vi "test1-ModuleCreatedDestroyed_Queue.vi"(8 "error in (no error)":errorcluster, 11 "TestCase in":refnum<class "testcase-CSMGlobalLog.lvclass">) -> (0 "error out":errorcluster, 3 "TestCase out":refnum<class "testcase-CSMGlobalLog.lvclass">)   [LabVIEW 2017, in "testcase-CSMGlobalLog.lvclass"]
uses:
  testcase-CSMGlobalLog.lvclass
  testcase-CSMGlobalLog.lvclass/testcase-CSMGlobalLog.ctl
  64b6e408-f0cd-4aee-a387-1a6bb95babb2.vi
  <vilib>/addons/_JKI Toolkits/VI Tester/TestCase.llb/TestCase.lvclass
  src/user.lib/_NEVSTOP/Communicable State Machine(CSM)/Utility/Periodic String Filter Setting.ctl
  src/user.lib/_NEVSTOP/Communicable State Machine(CSM)/Communicable State Machine.lvlib
  C:/Program Files (x86)/National Instruments/LabVIEW 2017/vi.lib/addons/_JKI Toolkits/VI Tester/TestCase.llb/TestCase.lvclass
panel:
  out "String Cache Each Loop":string
  out "String cache total":string
  out "LoopCount":i32
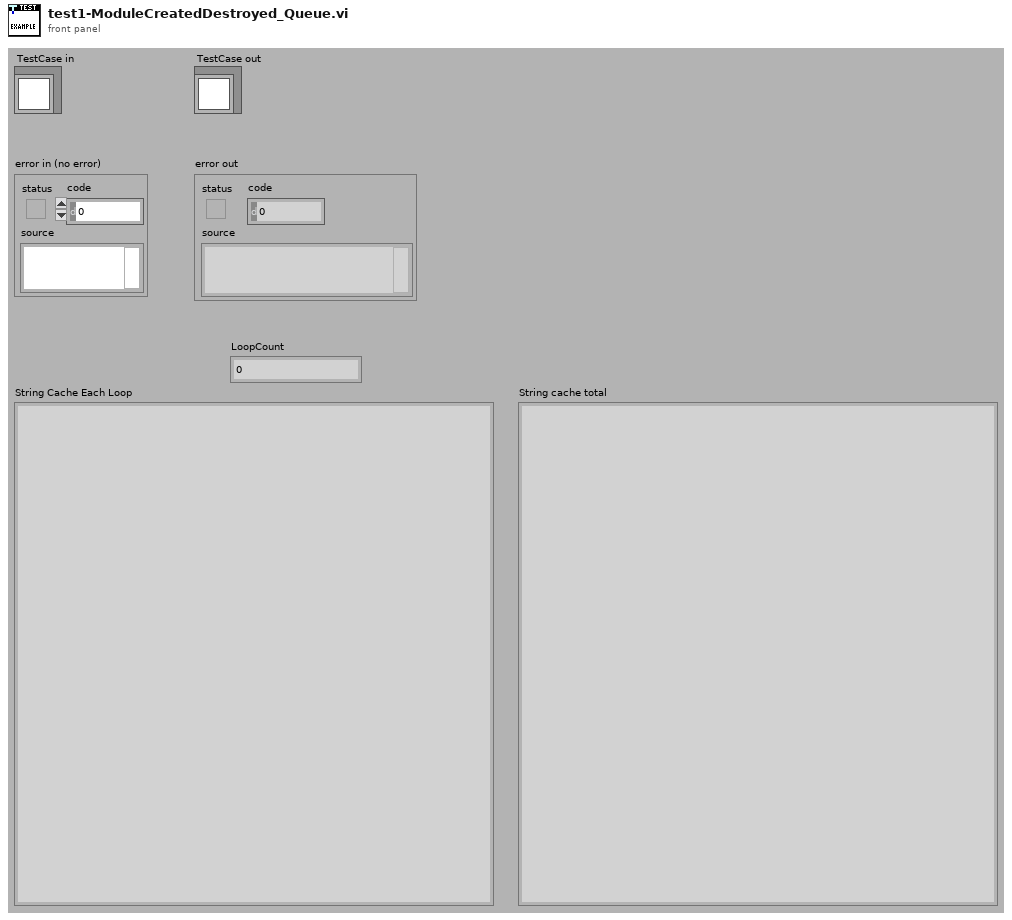
[diagram p1: front panel]
types:
  T1 = typedef "Communicable State Machine.lvlib/Periodic String Filter Setting.ctl" = cluster{"threashold(#/s)":dbl, "Check Peroid(s)":dbl}
  T2 = typedef "Communicable State Machine.lvlib/_CSM_GlobalLog_MSG.ctl" = cluster{"Name (\"\" to Use UUID)":string, "Current State":string, "Arguments":string, "Source Message":T3, "Source Module":string, "Complete(T)/Start(F)":bool, "LogType":T4, "Time Stamp":timestamp}
  T3 = typedef "Communicable State Machine.lvlib/_CSM_Response Source Message.ctl" = cluster{"‘State":string, "’Arguments":string, "’Error":errorcluster}
  T4 = typedef "Communicable State Machine.lvlib/_CSM_GlobalLog_MSG_TYPE.ctl" = enum16{"User Log", "State Change", "Status", "Interrupt", "Register", "Unregister", "Error Log", "Module Created", "Module Destroyed", "Async Message", "No-Rep Async Message", "Sync Message", "AsyncMsg Complete", "SyncMsg Complete"}
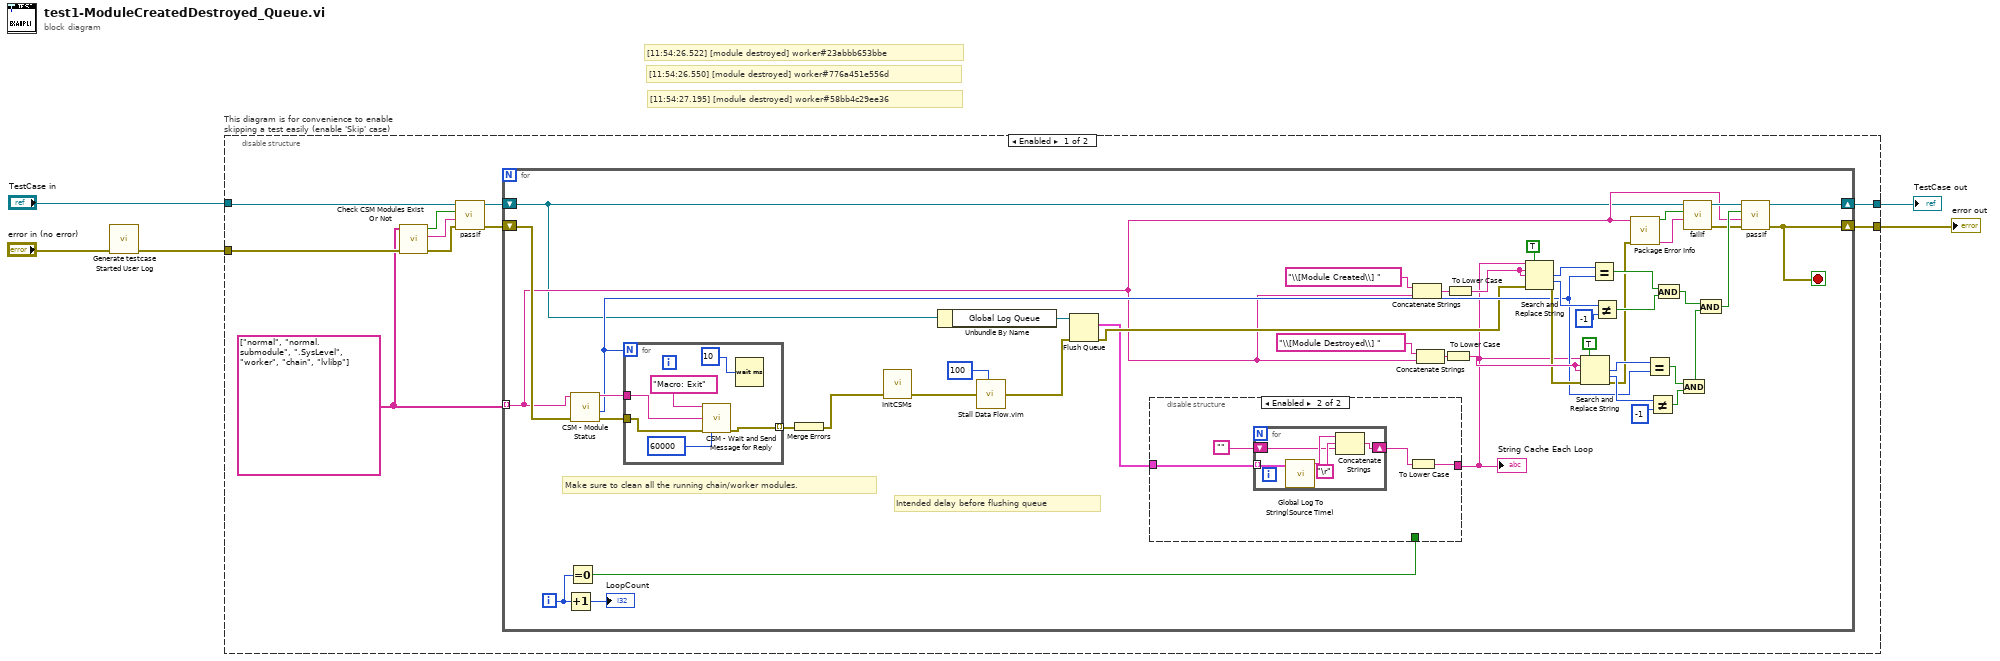
[diagram p0: block diagram]
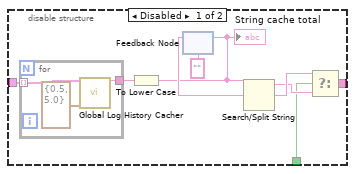
[diagram p2: hidden frame]
diagram:
  # "[11:54:26.522] [module destroyed] worker#23abbb653bbe"
  # "[11:54:27.195] [module destroyed] worker#58bb4c29ee36"
  # "[11:54:26.550] [module destroyed] worker#776a451e556d"
  n1 = call "Generate testcase Started User Log.vi"("Error In"="error in (no error)") -> ("error out"=w1:errorcluster)  [unwired: 10 in]
  n2 = disable-structure "This diagram is for convenience to enable skipping a test easily (enable 'Skip' case)" shown="Enabled" {
    disable-tunnel: "TestCase in" -> [w10 w93]
    disable-tunnel: [w14 w91] -> w2
    disable-tunnel: [w15 w92] -> w4
    disable-tunnel: w1 -> [w8 w90]
    frame Enabled {
      w6 = string[] ["normal", "normal.submodule", ".SysLevel", "worker", "chain", "lvlibp"]
      n3 = call "Check CSM Modules Exist Or Not.vi"("error in"=w8, "CSM names in"=w6) -> ("error out"=w11:errorcluster, "Debug string"=w12:string, "All Modules Exist?"=w13:bool)  [unwired: 7 in]
      n4 = call-dynamic "passIf.vi"("error in (no error)"=w11, "message (\"\")"=w12, "pass"=w13, "TestCase in"=w10) -> ("error out"=w7:errorcluster, "TestCase out"=w9:refnum<class "testcase-CSMGlobalLog.lvclass">)  [unwired: 6 in]
      n5 = for {
        tunnel: w6 -> [w17] mode=indexing
        shift-right: [w32] -> w15
        shift-left: w7 -> [w24]
        shift-right: [w62] -> w14
        shift-left: w9 -> [w16]
        i -> [w26]
        stop <- w32 stop-if-true
        # "Intended delay before flushing queue"
        # "Make sure to clean all the running chain/worker modules."
        n6 = Increment(x=w26) -> (x+1=→"LoopCount":i32)
        n7 = Equal To 0?(x=w26) -> (x = 0?=w25:bool)
        n8 = call "CSM - Module Status.vi"("Error In"=w24, "CSM Name"=w17) -> ("error out"=w23:errorcluster, "#Nodes"=w38:i32, "CSM Name (Dup)"=w55:string)  [unwired: 5 in, 2 out]
        n9 = for {
          N: w38 -> [_]
          tunnel: [w88] -> w54 mode=indexing
          tunnel: w55 -> [w87]
          tunnel: w23 -> [w86]
          n10 = call "CSM - Wait and Send Message for Reply.vi"("State"="Macro: Exit", "Target Module"=w87, "Error In (No Error)"=w86, "Response Timeout (-2 Using Global Settings)"=60000) -> ("error out"=w88:errorcluster)  [unwired: 8 in, 3 out]
          n11 = Wait (ms)(milliseconds to wait=u32 10) -> ()  [unwired: 1 out]
        }
        n12 = Merge Errors(w54) -> (w33:errorcluster)
        n13 = call "InitCSMs.vi"("error in"=w33) -> ("error out"=w31:errorcluster)  [unwired: 9 in, 1 out]
        n14 = Unbundle By Name(w16) -> ("Global Log Queue"=w61:refnum<queue>)
        n15 = call "Stall Data Flow.vim"("value in"=w31, "milliseconds to wait"=u32 100) -> ("value out"=w30:errorcluster)  [unwired: 1 out]
        n16 = Flush Queue(queue=w61, error in (no error)=w30) -> (remaining elements=w28:T2[], error out=w34:errorcluster)  [unwired: 1 out]
        n17 = disable-structure shown="Enabled" {
          disable-tunnel: [w65 w75] -> w27
          disable-tunnel: w25 -> [w64 _]
          disable-tunnel: w28 -> [w63 w77]
          frame Disabled {
            n18 = for {
              tunnel: w63 -> [w74] mode=indexing
              tunnel: [w73] -> w71
              n19 = call "Global Log History Cacher.vi"("Global Log Data"=w74, "Settings"=T1 {"threashold(#/s)"=0.5, "Check Peroid(s)"=5.0}) -> ("String Cache"=w73:string)  [unwired: 13 in]
            }
            n20 = To Lower Case(string=w71) -> (all lower case string=w66:string)
            "String cache total" <- w66
            n21 = feedback #1("") -> (w70:string)
            n22 = feedback-in #1(w66) -> ()
            n23 = Search/Split String(string=w66, search string/char (-)=w70) -> (substring before match=w67:string, match + rest of string=w68:string)  [unwired: 1 in, 1 out]
            n24 = Select(t=w68, s=w64, f=w67) -> (s? t:f=w65:string)
          }
          frame Enabled {
            n25 = for {
              tunnel: w77 -> [w83] mode=indexing
              shift-right: [w79] -> w76
              shift-left: "" -> [w80]
              n26 = call "Global Log To String(Source Time).vi"("Log"=w83) -> ("Log String"=w82:string)  [unwired: 9 in]
              n27 = Concatenate Strings(w82, "\r", w80) -> (w79:string)
            }
            n28 = To Lower Case(string=w76) -> (all lower case string=w75:string)
          }
        }
        "String Cache Each Loop" <- w27
        n29 = Concatenate Strings("\\[Module Created\\] " ("regular expression"), w17) -> (w56:string)
        n30 = Concatenate Strings("\\[Module Destroyed\\] " ("regular expression"), w17) -> (w58:string)
        n31 = To Lower Case(string=w58) -> (all lower case string=w40:string)
        n32 = To Lower Case(string=w56) -> (all lower case string=w52:string)
        n33 = Search and Replace String(replace all?=TRUE ("replace all? (F)"), input string=w27, search string=w52, replace string=w52, error in=w34) -> (number of replacements=w51:i32, offset past replacement=w50:i32, error out=w39:errorcluster)  [unwired: 3 in, 1 out]
        n34 = Search and Replace String(replace all?=TRUE ("replace all? (F)"), input string=w27, search string=w40, replace string=w40, error in=w39) -> (number of replacements=w42:i32, offset past replacement=w43:i32, error out=w18:errorcluster)  [unwired: 3 in, 1 out]
        n35 = Equal?(x=w51, y=w38) -> (x = y?=w48:bool)
        n36 = Not Equal?(x=w50, y=-1) -> (x != y?=w47:bool)
        n37 = call "Package Error Info.vi"("error in"=w18, "String in"=w17) -> ("packed error info out"=w21:string, "error status"=w22:bool)  [unwired: 8 in]
        n38 = Equal?(x=w42, y=w38) -> (x = y?=w45:bool)
        n39 = Not Equal?(x=w43, y=-1) -> (x != y?=w46:bool)
        n40 = And(x=w48, y=w47) -> (x .and. y?=w37:bool)
        n41 = And(x=w45, y=w46) -> (x .and. y?=w36:bool)
        n42 = call-dynamic "failIf.vi"("message (\"\")"=w21, "fail"=w22, "TestCase in"=w16) -> ("error out"=w19:errorcluster, "TestCase out"=w20:refnum<class "testcase-CSMGlobalLog.lvclass">)  [unwired: 7 in]
        n43 = And(x=w37, y=w36) -> (x .and. y?=w35:bool)
        n44 = call-dynamic "passIf.vi"("error in (no error)"=w19, "message (\"\")"=w17, "pass"=w35, "TestCase in"=w20) -> ("error out"=w32:errorcluster, "TestCase out"=w62:refnum<class "testcase-CSMGlobalLog.lvclass">)  [unwired: 6 in]
      }
    }
    frame Disabled {
      # "skip test result while test is under development"
      n45 = call <vilib>:"skip.vi"("error in (no error)"=w90, "TestCase in"=w93) -> ("error out"=w92:errorcluster, "TestCase out"=w91:refnum<class "testcase-CSMGlobalLog.lvclass">)  [unwired: 8 in]
    }
  }
  "error out" <- w4
  "TestCase out" <- w2
